vi "Read Bid.vi"(8 "error in (no error)":errorcluster, 11 "Hand in":refnum<class "Hand.lvclass">) -> (0 "error out":errorcluster, 2 "Bid":u64, 3 "Hand out":refnum<class "Hand.lvclass">)   [LabVIEW 2020, in "Hand.lvclass"]
uses:
  Hand.lvclass
  Hand.lvclass/Hand.ctl
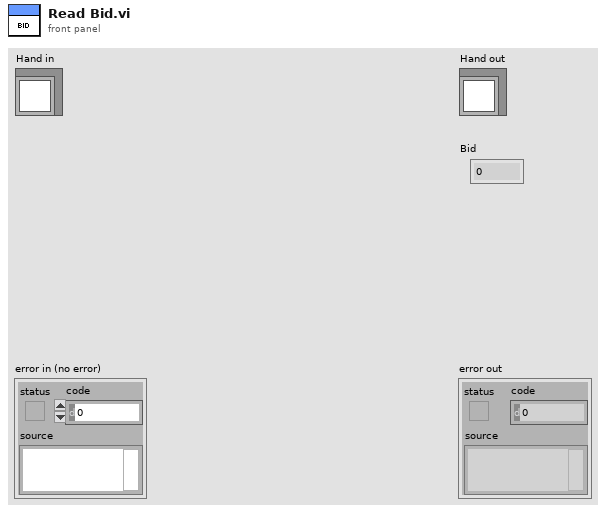
[diagram p1: front panel]
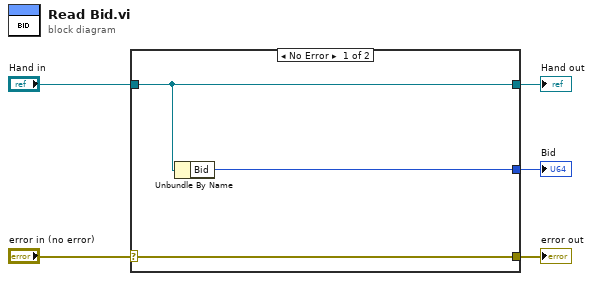
[diagram p0: block diagram]
diagram:
  n1 = case shown="No Error" "error in (no error)" {
    selector: "error in (no error)" -> [w8 w9]
    tunnel: [w8 w9] -> w4
    tunnel: [w7 w10] -> w2
    tunnel: "Hand in" -> [w7 w10]
    tunnel: [w6 _] -> w1
    frame No Error {
      n2 = Unbundle By Name(w7) -> ("Bid"=w6:u64)
    }
    frame Error {
    }
  }
  "error out" <- w4
  "Hand out" <- w2
  "Bid" <- w1
